vi "BatteryCharge.vi"() -> ()   [LabVIEW 2021]
panel:
  in  "array":dbl[](array[numeric])
  in  "Numeric":dbl=0.692 min=0.692 max=1.506 step=0.05 format="%#_13g"
  in  "Stop":bool
  out "Battery Percentage":dbl caption="%" format="%#_2g%%"
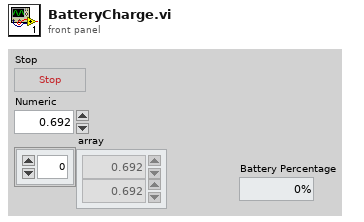
[diagram p1: front panel]
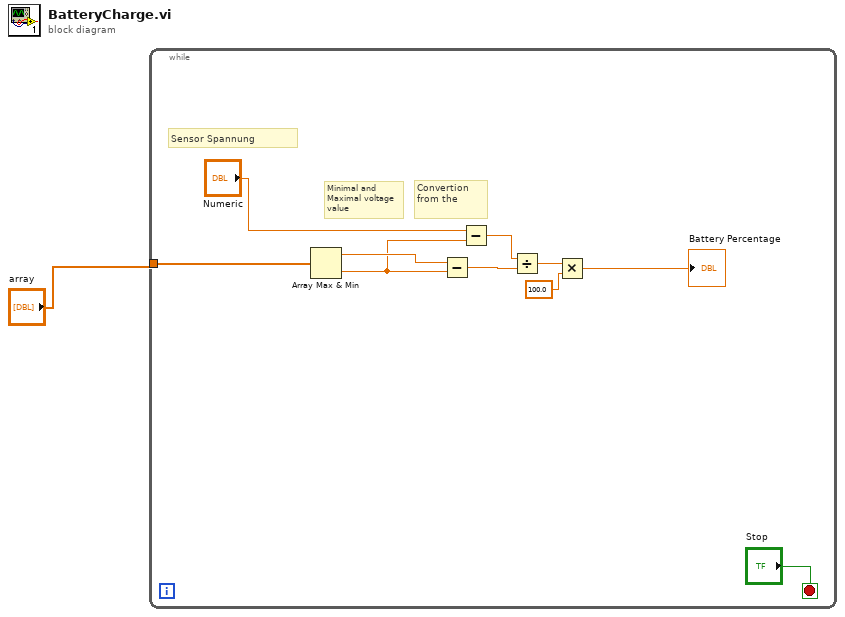
[diagram p0: block diagram]
diagram:
  n1 = while {
    tunnel: "array" -> [w4]
    stop <- "Stop" stop-if-true
    # "Sensor Spannung"
    # "Convertion \nfrom the"
    # "Minimal and \nMaximal voltage\nvalue"
    n2 = Array Max & Min(array=w4) -> (max value=w11:dbl, min value=w9:dbl)  [unwired: 2 out]
    n3 = Subtract(x=w11, y=w9) -> (x-y=w10:dbl)
    n4 = Subtract(x="Numeric", y=w9) -> (x-y=w8:dbl)
    n5 = Divide(x=w8, y=w10) -> (x/y=w7:dbl)
    n6 = Multiply(x=w7, y=100.0) -> (x*y=→"Battery Percentage":dbl)
  }
